vi "Get Configuration Cluster.vi"(8 "error in (no error)":errorcluster, 11 "Plugin Configuration in":refnum<class "Plugin Configuration.lvclass">) -> (0 "error out":errorcluster, 2 "plugin configuration":T1={"core"={"name"="", "components"=[], "cycle timing"={"priority"=10000, "decimation"=1, "offset"=0}}, "component settings"=[], "threads"=[]}, 3 "Plugin Configuration out":refnum<class "Plugin Configuration.lvclass">)   [LabVIEW 2019, in "DSF Core.lvlib" / "Plugin Configuration.lvclass"]
uses:
  Plugin Configuration.lvclass
  C:/Dev/GitHub/niveristand-data-sharing-framework-custom-device/Core/Classes/Configuration/Core/Core Configuration.lvclass
  Typedefs/DSF Engine Plugin Configuration.ctl
  Typedefs/Core Plugin Configuration.ctl
  Typedefs/DSF Timing Info.ctl
  Typedefs/DSF Settings Info.ctl
  Typedefs/DSF Engine Plugin Thread Configuration.ctl
  Typedefs/Core Thread Configuration.ctl
  Typedefs/DSF Engine Transfer Group Configuration.ctl
  Typedefs/Core Group Configuration.ctl
  Typedefs/DSF Direction.ctl
  Typedefs/DSF Timeout Behavior.ctl
  Typedefs/DSF Engine Transfer Configuration.ctl
  Typedefs/Core Transfer Configuration.ctl
  Typedefs/DSF Engine Channel Configuration.ctl
  Typedefs/Core Channel Configuration.ctl
  Typedefs/DSF Data Type.ctl
  Core Configuration.lvclass/Core Configuration.ctl
  Plugin Configuration.lvclass/Plugin Configuration.ctl
  Thread/Thread Configuration.lvclass/Thread Configuration.ctl
  Group/Group Configuration.lvclass/Group Configuration.ctl
  Transfer/Transfer Configuration.lvclass/Transfer Configuration.ctl
  Thread/Thread Configuration.lvclass
  Group/Group Configuration.lvclass
  Transfer/Transfer Configuration.lvclass
  DSF Core.lvlib
  Core Configuration.lvclass
  Channel/Channel Configuration.lvclass
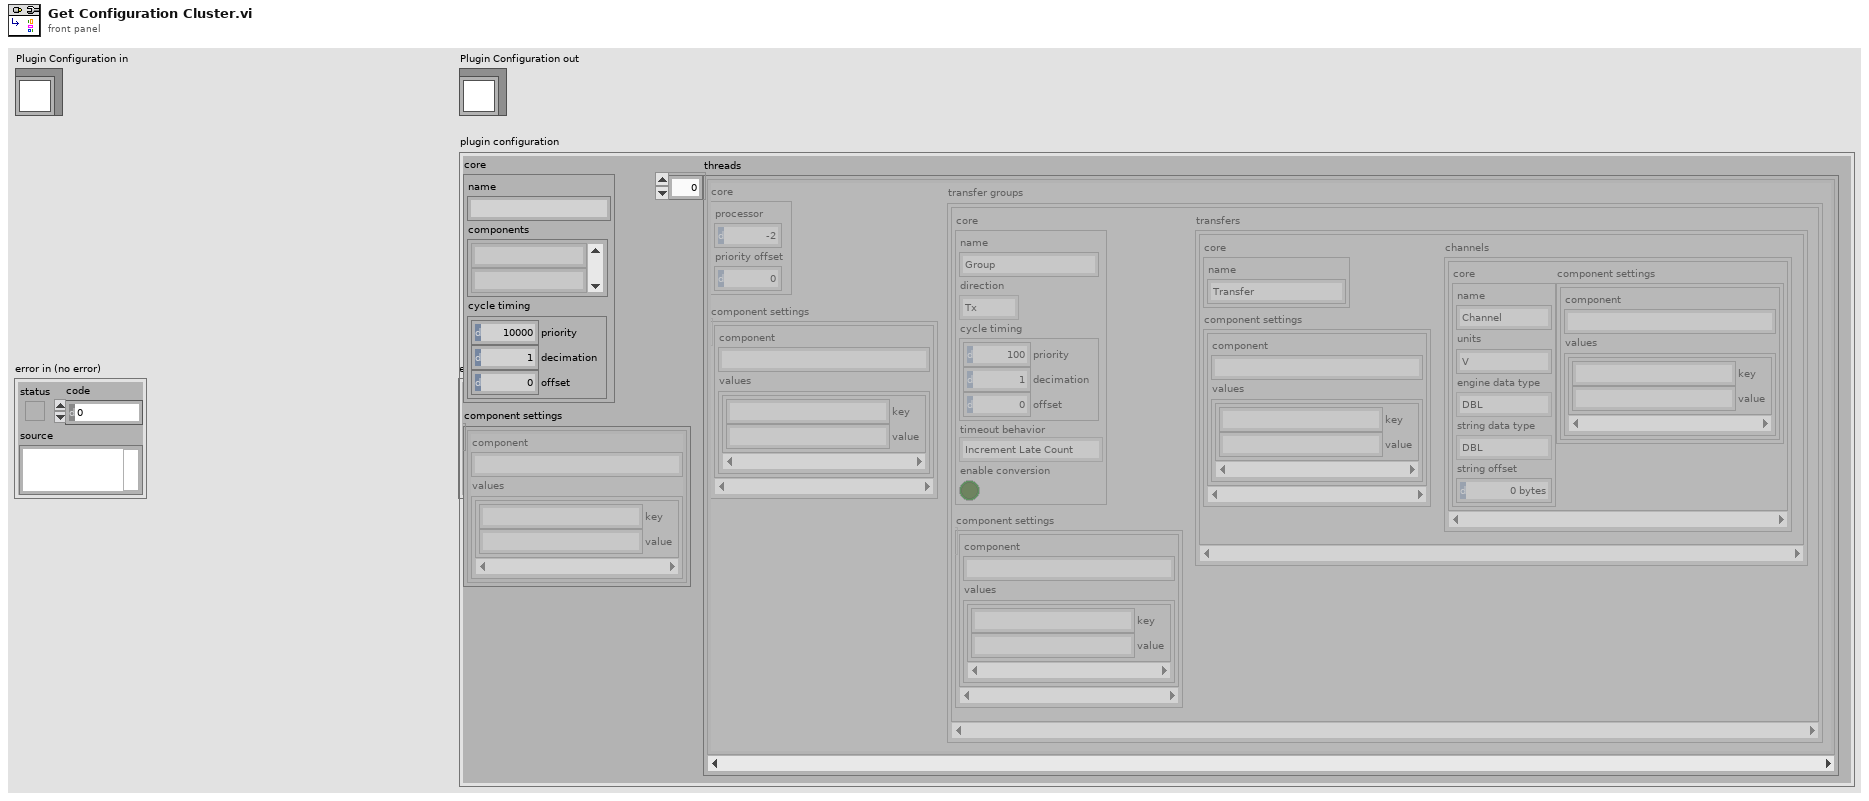
[diagram p1: front panel]
types:
  T1 = typedef "DSF Core.lvlib/DSF Engine Plugin Configuration.ctl" = cluster{"core":T2, "component settings":T4[], "threads":T5[]}
  T2 = typedef "DSF Core.lvlib/Plugin Configuration.lvclass/Core Plugin Configuration.ctl" = cluster{"name":string, "components":string[], "cycle timing":T3}
  T3 = typedef "DSF Core.lvlib/DSF Timing Info.ctl" = cluster{"priority":u64, "decimation":u64, "offset":u64}
  T4 = typedef "DSF Core.lvlib/DSF Settings Info.ctl" = cluster{"component":string, "values":cluster{"key":string, "value":string}[]}
  T5 = typedef "DSF Core.lvlib/DSF Engine Plugin Thread Configuration.ctl" = cluster{"core":T6, "component settings":T4[], "transfer groups":T7[]}
  T6 = typedef "DSF Core.lvlib/Thread Configuration.lvclass/Core Thread Configuration.ctl" = cluster{"processor":i32, "priority offset":i16}
  T7 = typedef "DSF Core.lvlib/DSF Engine Transfer Group Configuration.ctl" = cluster{"core":T8, "component settings":T4[], "transfers":T11[]}
  T8 = typedef "DSF Core.lvlib/Group Configuration.lvclass/Core Group Configuration.ctl" = cluster{"name":string, "direction":T9, "cycle timing":T3, "timeout behavior":T10, "enable conversion":bool}
  T9 = typedef "DSF Core.lvlib/DSF Direction.ctl" = enum8{"Tx", "Rx"}
  T10 = typedef "DSF Core.lvlib/DSF Timeout Behavior.ctl" = enum8{"Increment Late Count", "Throw Error"}
  T11 = typedef "DSF Core.lvlib/DSF Engine Transfer Configuration.ctl" = cluster{"core":T12, "component settings":T4[], "channels":T13[]}
  T12 = typedef "DSF Core.lvlib/Transfer Configuration.lvclass/Core Transfer Configuration.ctl" = cluster{"name":string}
  T13 = typedef "DSF Core.lvlib/DSF Engine Channel Configuration.ctl" = cluster{"core":T14, "component settings":T4[]}
  T14 = typedef "DSF Core.lvlib/Channel Configuration.lvclass/Core Channel Configuration.ctl" = cluster{"name":string, "units":string, "engine data type":T15, "string data type":T15, "string offset":u64}
  T15 = typedef "DSF Core.lvlib/DSF Data Type.ctl" = enum8{"Bool", "SGL", "DBL", "I8", "I16", "I32", "I64", "U8", "U16", "U32", "U64"}
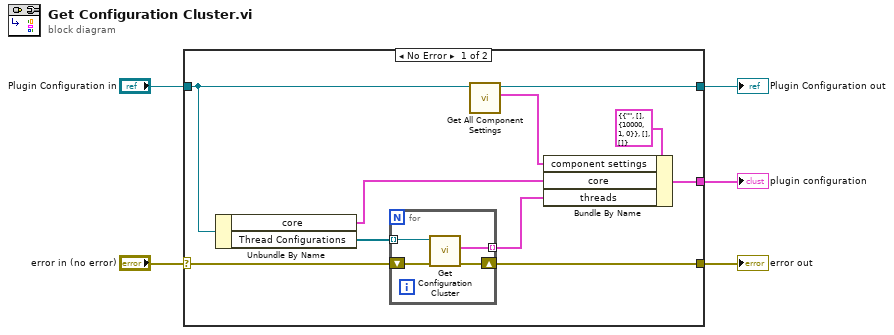
[diagram p0: block diagram]
diagram:
  n1 = case shown="No Error" "error in (no error)" {
    selector: "error in (no error)" -> [w15 w21]
    tunnel: [w14 w21] -> w4
    tunnel: [w8 w20] -> w2
    tunnel: "Plugin Configuration in" -> [w7 w20]
    tunnel: [w10 _] -> w1
    frame No Error {
      n2 = Unbundle By Name(w7) -> ("core"=w6:T2, "Thread Configurations"=w12:refnum<class "Thread Configuration.lvclass">[])
      n3 = for {
        shift-right: [w18] -> w14
        shift-left: w15 -> [w19]
        tunnel: [w16] -> w13 mode=indexing
        tunnel: w12 -> [w17] mode=indexing
        n4 = call "Get Configuration Cluster.vi"("error in (no error)"=w19, "Thread Configuration in"=w17) -> ("error out"=w18:errorcluster, "thread configuration"=w16:T5)  [unwired: 7 in, 1 out]
      }
      n5 = call "Get All Component Settings.vi"("Runtime Configuration in"=w7) -> ("component settings"=w9:T4[], "Runtime Configuration out"=w8:refnum<class "Plugin Configuration.lvclass">)  [unwired: 8 in, 1 out]
      n6 = Bundle By Name(cluster=T1 {"core"={"name"="", "components"=[], "cycle timing"={"priority"=10000, "decimation"=1, "offset"=0}}, "component settings"=[], "threads"=[]} ("plugin configuration"), "component settings"=w9, "core"=w6, "threads"=w13) -> (w10:T1)
    }
    frame Error {
    }
  }
  "error out" <- w4
  "Plugin Configuration out" <- w2
  "plugin configuration" <- w1
